vi "DAQ-GetTimeControlParameters.vi"(3 "tiempo (ms)":dbl, 5 "DAQ Device IN":T1) -> (1 "#samples":u32, 2 "Time Control Parameters":cluster{"# samples":u32, "tiempos (ms)":dbl})   [LabVIEW 2010]
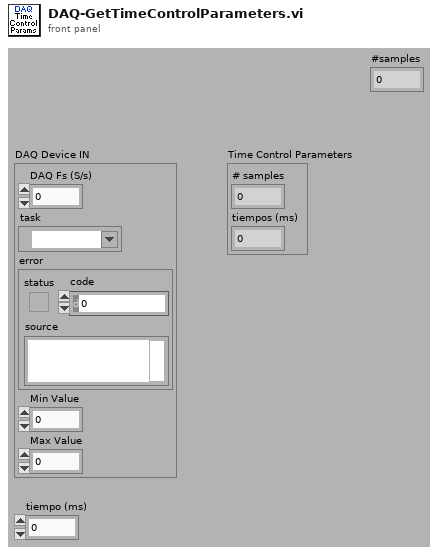
[diagram p1: front panel]
types:
  T1 = cluster{"DAQ Fs (S/s)":dbl, "task":refnum<k21>, "error":errorcluster, "Min Value":dbl, "Max Value":dbl}
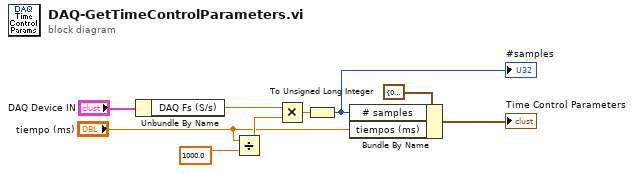
[diagram p0: block diagram]
diagram:
  n1 = Unbundle By Name("DAQ Device IN") -> ("DAQ Fs (S/s)"=w9:dbl)
  n2 = Divide(x="tiempo (ms)", y=sgl 1000.0) -> (x/y=w2:dbl)
  n3 = Multiply(x=w9, y=w2) -> (x*y=w6:dbl)
  n4 = To Unsigned Long Integer(number=w6) -> (unsigned 32bit integer=w7:u32)
  "#samples" <- w7
  n5 = Bundle By Name(cluster=cluster{"# samples":u32, "tiempos (ms)":dbl} {"# samples"=0, "tiempos (ms)"=0.0} ("Time Control Parameters"), "# samples"=w7, "tiempos (ms)"="tiempo (ms)") -> (→"Time Control Parameters":cluster{"# samples":u32, "tiempos (ms)":dbl})
